vi "20211001_HW00.vi"() -> ()   [LabVIEW 2019]
panel:
  in  "ShowChg.Btn.Color":bool
  in  "Changed Colors":cluster{"Color Box":u32, "Color Box 2":u32}[](array[cluster])=[{"Color Box"=16777216, "Color Box 2"=16777216}, {"Color Box"=16711680, "Color Box 2"=16711680}, {"Color Box"=16777216, "Color Box 2"=16777216}, {"Color Box"=4424887, "Color Box 2"=4424887}]
  in  "Original Colors":cluster{"Color Box":u32, "Color Box 2":u32}[](array[cluster])=[{"Color Box"=16777216, "Color Box 2"=16777216}, {"Color Box"=4424887, "Color Box 2"=4424887}, {"Color Box"=16777216, "Color Box 2"=16777216}, {"Color Box"=4424887, "Color Box 2"=4424887}]
  in  "Chg.Btn.Color":bool
  in  "Button":bool
  # "Press \"Home\" key on keyboard can toggle this button."
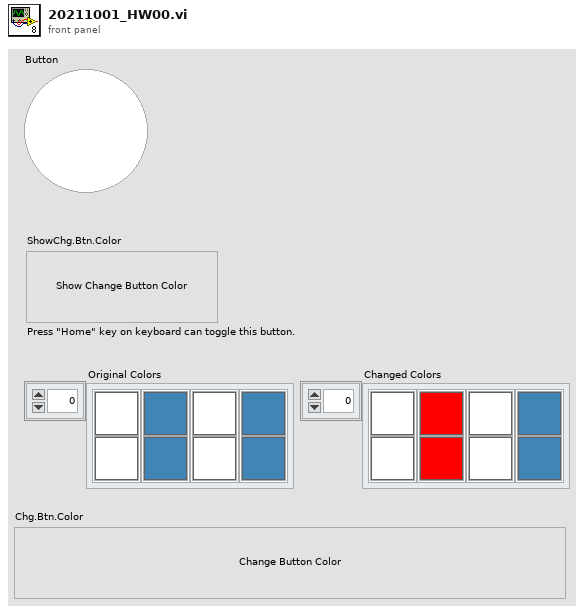
[diagram p1: front panel]
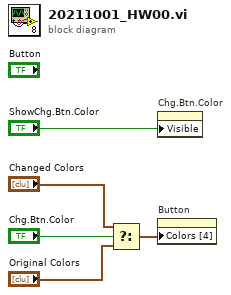
[diagram p0: block diagram]
diagram:
  n1 = Select(t="Changed Colors", s="Chg.Btn.Color", f="Original Colors") -> (s? t:f=w1:cluster{"Color Box":u32, "Color Box 2":u32}[])
  n2 = property on="Chg.Btn.Color" class="Bool (strict)"("Visible"="ShowChg.Btn.Color") -> ()  [unwired: 2 in, 2 out]
  n3 = property on="Button" class="Bool (strict)"("Colors [4]"=w1) -> ()  [unwired: 2 in, 2 out]
